vi "DateTime.vi"() -> ()   [LabVIEW 2013]
doc: "This VI demostrated conver datetime string to timestamp"
uses:
  <vilib>/Utility/miscctls.llb/LVDateTimeRec.ctl
panel:
  out "time stamp":timestamp
  out "demostrate date time string":string
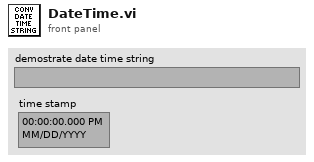
[diagram p1: front panel]
types:
  T1 = typedef "LVDateTimeRec.ctl" = cluster{"fractional second":dbl, "second":i32, "minute":i32, "hour":i32, "day of month":i32, "month":i32, "year":i32, "day of week":i32, "day of year":i32, "DST":i32}
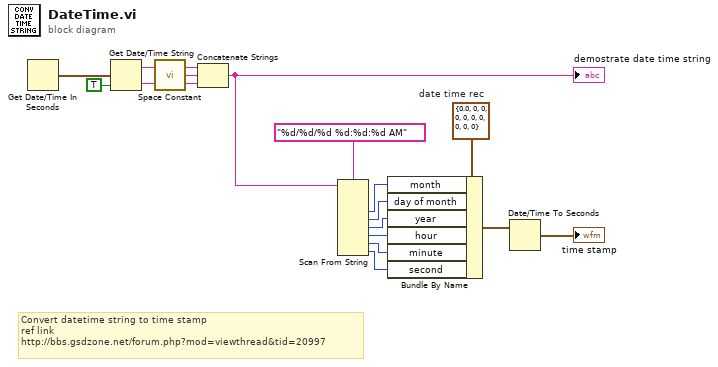
[diagram p0: block diagram]
diagram:
  w11 = T1 {"fractional second"=0.0, "second"=0, "minute"=0, "hour"=0, "day of month"=0, "month"=0, "year"=0, "day of week"=0, "day of year"=0, "DST"=0}  # date time rec
  # "Convert datetime string to time stamp\nref link\nhttp://bbs.gsdzone.net/forum.php?mod=viewthread&tid=20997"
  n1 = Get Date/Time In Seconds() -> (seconds since 1Jan1904=w16:timestamp)
  n2 = Get Date/Time String(seconds (now)=w16, want seconds? (F)=TRUE) -> (date string=w14:string, time string=w12:string)  [unwired: 1 in]
  n3 = call <vilib>:"Space Constant.vi"() -> ("String"=w13:string)
  n4 = Concatenate Strings(w14, w13, w12) -> (w8:string)
  "demostrate date time string" <- w8
  n5 = Scan From String(format string="%d/%d/%d %d:%d:%d AM", input string=w8) -> (output 1=w6:i32, output 2=w5:i32, output 3=w4:i32, output 4=w3:i32, output 5=w2:i32, output 6=w1:i32)  [unwired: 8 in, 3 out]
  n6 = Bundle By Name(cluster=w11, "month"=w6, "day of month"=w5, "year"=w4, "hour"=w3, "minute"=w2, "second"=w1) -> (w10:T1)
  n7 = Date/Time To Seconds(2:w10) -> (0:→"time stamp":timestamp)  [unwired: 1 in]
